vi "Open Office File.vi"(11 "Selection a Word (.doc, .docx), Excel (.xls, .xlsx), or Powerpoint (.ppt, .pptx) Document...":path) -> (3 "error out":errorcluster)   [LabVIEW 2019]
uses:
  <vilib>/registry/registry.llb/Read Registry Value Simple STR.vi
  <vilib>/registry/registry.llb/Registry RtKey.ctl
  <vilib>/registry/registry.llb/Registry SAM.ctl
  <vilib>/registry/registry.llb/Registry View.ctl
panel:
  out "File Dialog Cancelled?":bool
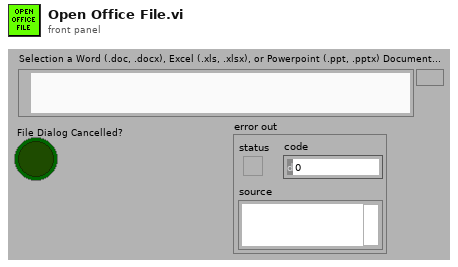
[diagram p1: front panel]
types:
  T1 = typedef "Registry SAM.ctl" = enum32{"KEY_QUERY_VALUE", "KEY_SET_VALUE", "KEY_CREATE_SUB_KEY", "KEY_ENUMERATE_SUB_KEYS", "KEY_NOTIFY", "KEY_CREATE_LINK", "KEY_READ", "KEY_WRITE", "KEY_ALL_ACCESS", "KEY_READ | KEY_WRITE"}
  T2 = typedef "Registry RtKey.ctl" = enum32{"HKEY_CLASSES_ROOT", "HKEY_CURRENT_USER", "HKEY_LOCAL_MACHINE", "HKEY_USERS", "HKEY_PERFORMANCE_DATA", "HKEY_CURRENT_CONFIG", "HKEY_DYN_DATA"}
  T3 = typedef "Registry View.ctl" = u16
  T4 = typedef "Registry refnum.ctl" = refnum<k1>
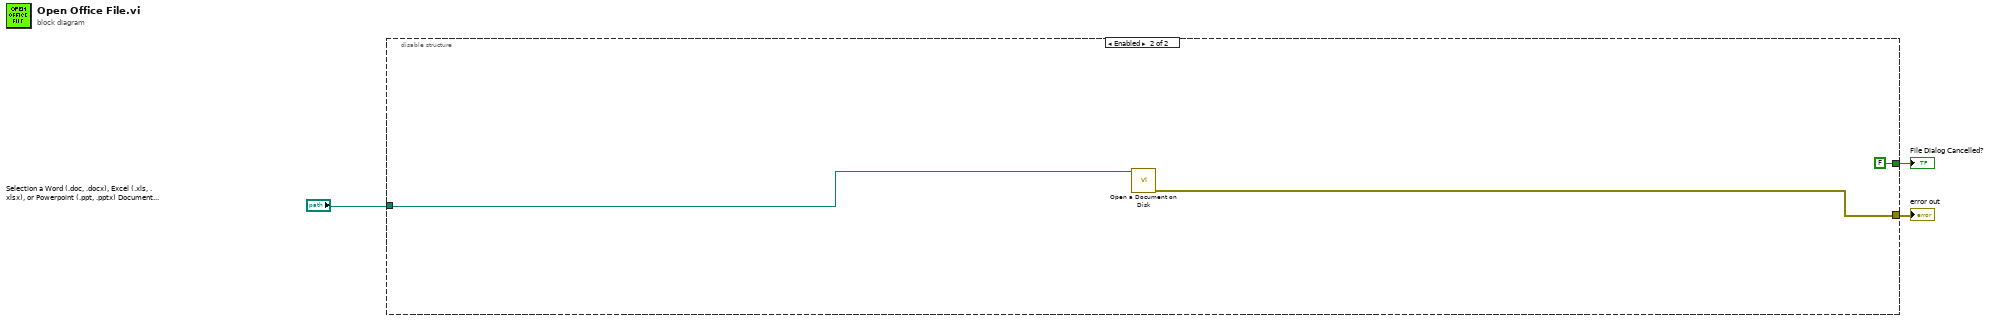
[diagram p0: block diagram]
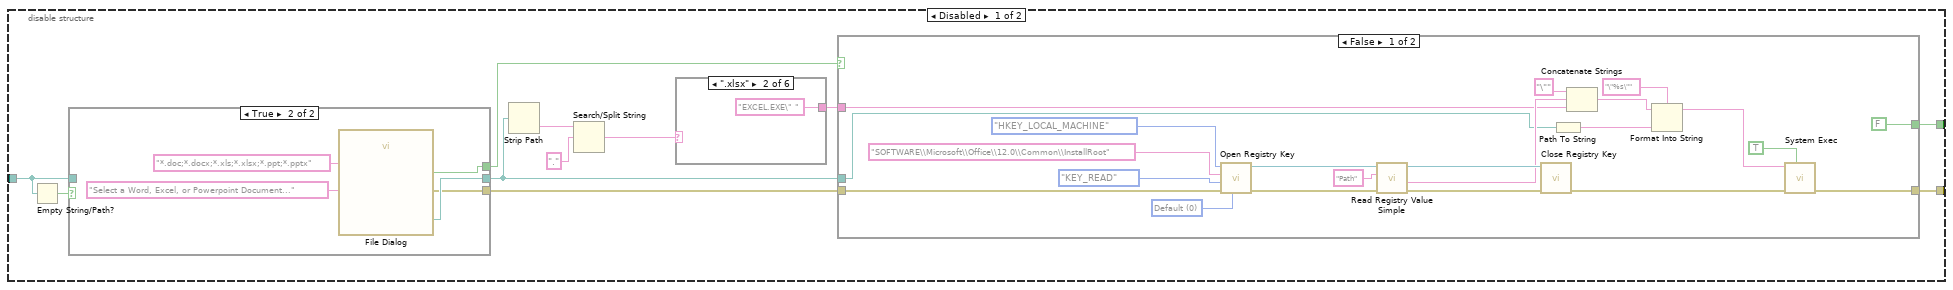
[diagram p2: hidden frame]
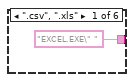
[diagram p3: hidden frame]
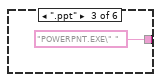
[diagram p4: hidden frame]
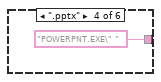
[diagram p5: hidden frame]
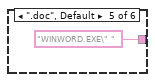
[diagram p6: hidden frame]
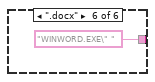
[diagram p7: hidden frame]
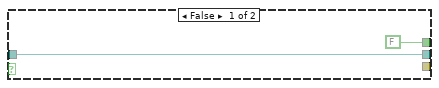
[diagram p8: hidden frame]
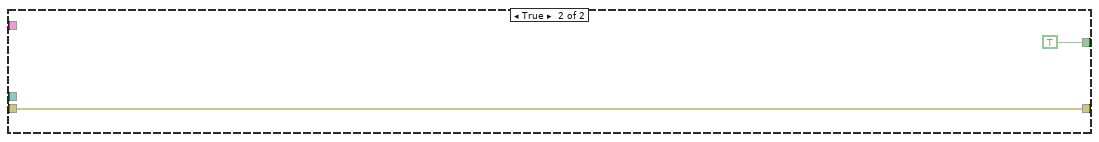
[diagram p9: hidden frame]
diagram:
  n1 = disable-structure shown="Enabled" {
    disable-tunnel: [w14 FALSE ("File Dialog Cancelled?")] -> w3
    disable-tunnel: "Selection a Word (.doc, .docx), Excel (.xls, .xlsx), or Powerpoint (.ppt, .pptx) Document..." -> [w12 w52]
    disable-tunnel: [w4 w54] -> w1
    frame Disabled {
      n2 = Empty String/Path?(string/path=w12) -> (empty?=w13:bool)
      n3 = case shown="True" w13 {
        tunnel: [FALSE ("cancelled") w25] -> w11
        tunnel: [w22 w24] -> w5
        tunnel: w12 -> [w22 _]
        tunnel: [_ w23] -> w10
        frame False {
        }
        frame True {
          n4 = call "File Dialog"("prompt"="Select a Word, Excel, or Powerpoint Document...", "pattern (all files)"="*.doc;*.docx;*.xls;*.xlsx;*.ppt;*.pptx") -> ("selected path"=w24:path, "cancelled"=w25:bool, "error out"=w23:errorcluster)  [unwired: 10 in, 1 out]
        }
      }
      n5 = Strip Path(path=w5) -> (name=w9:string)  [unwired: 1 out]
      n6 = Search/Split String(string=w9, search string/char (-)=".") -> (match + rest of string=w7:string)  [unwired: 1 in, 2 out]
      n7 = case shown="\".xlsx\"" w7 {
        tunnel: ["EXCEL.EXE\" " "EXCEL.EXE\" " "POWERPNT.EXE\" " "POWERPNT.EXE\" " "WINWORD.EXE\" " "WINWORD.EXE\" "] -> w6
        frame ".csv", ".xls" {
        }
        frame ".xlsx" {
        }
        frame ".ppt" {
        }
        frame ".pptx" {
        }
        frame ".doc", Default {
        }
        frame ".docx" {
        }
      }
      n8 = case shown="False" w11 {
        tunnel: w10 -> [w37 w51]
        tunnel: [w28 w51] -> w4
        tunnel: [FALSE TRUE] -> w14
        tunnel: w6 -> [w31 _]
        tunnel: w5 -> [w30 _]
        frame False {
          w42 = T3 0 items=["Default"=0, "KEY_WOW64_64KEY"=8, "KEY_WOW64_32KEY"=9] ("registry view")
          n9 = call <vilib>:"Open Registry Key.vi"("registry view"=w42, "error in (no error)"=w37, "security access mask (KEY_READ | KEY_WRITE)"=Registry_SAM."KEY_READ", "subkey"="SOFTWARE\\Microsoft\\Office\\12.0\\Common\\InstallRoot", "root key (HKEY_LOCAL_MACHINE)"=Registry_RtKey."HKEY_LOCAL_MACHINE") -> ("error out"=w47:errorcluster, "refnum out"=w49:T4)  [unwired: 5 in]
          n10 = call-poly <vilib>:"Read Registry Value Simple.vi"("error in (no error)"=w47, "value"="Path", "refnum"=w49) -> ("error out"=w46:errorcluster, "String/Binary data"=w38:string, "refnum out"=w48:T4)  [unwired: 3 in, 1 out]
          n11 = call <vilib>:"Close Registry Key.vi"("error in (no error)"=w46, "refnum"=w48) -> ("error out"=w29:errorcluster)  [unwired: 5 in]
          n12 = Path To String(path=w30) -> (string=w39:string)
          n13 = Concatenate Strings("\"" ("string"), w38, w31) -> (w32:string)
          n14 = Format Into String "Format Into String"(format string="\"%s\"", initial string=w32, w39) -> (resulting string=w35:string)  [unwired: 1 in, 1 out]
          n15 = call <vilib>:"System Exec.vi"("wait until completion? (T)"=TRUE, "error in (no error)"=w29, "command line"=w35) -> ("error out"=w28:errorcluster)  [unwired: 5 in, 3 out]
        }
        frame True {
        }
      }
    }
    frame Enabled {
      n16 = call <vilib>:"Open a Document on Disk.vi"("document path"=w52) -> ("error out"=w54:errorcluster)  [unwired: 6 in]
    }
  }
  "File Dialog Cancelled?" <- w3
  "error out" <- w1
